vi "test_TCP_TCP Get Error Node.vi"(8 "error in (no error)":errorcluster, 11 "TestCase in":refnum<class "Ethernet Protocol Tests.lvclass">) -> (0 "error out":errorcluster, 3 "TestCase out":refnum<class "Ethernet Protocol Tests.lvclass">)   [LabVIEW 2019, in "Ethernet Protocol Tests.lvclass"]
uses:
  Ethernet Protocol Tests.lvclass
  TCP/TCP.lvclass
  <vilib>/addons/_JKI Toolkits/VI Tester/TestCase.llb/TestCase.lvclass
  C:/Program Files (x86)/National Instruments/LabVIEW 2019/vi.lib/addons/_JKI Toolkits/VI Tester/TestCase.llb/TestCase.lvclass
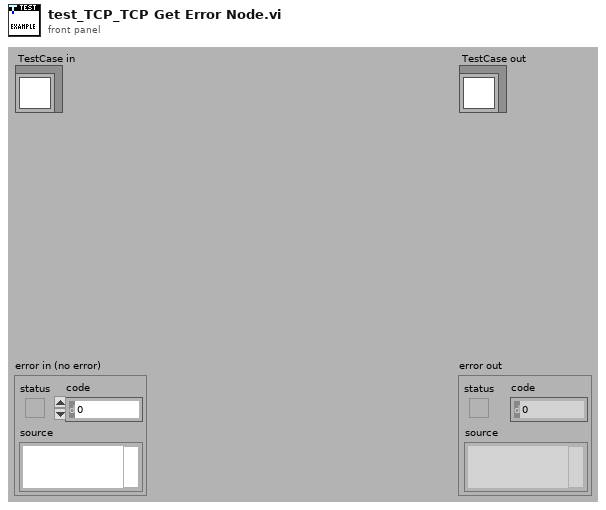
[diagram p1: front panel]
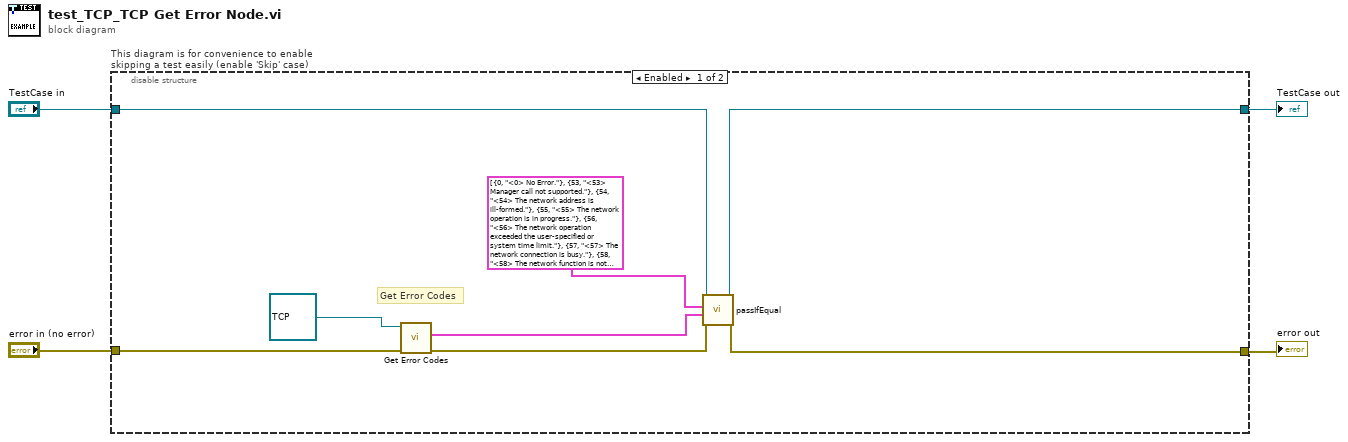
[diagram p0: block diagram]
diagram:
  n1 = disable-structure "This diagram is for convenience to enable skipping a test easily (enable 'Skip' case)" shown="Enabled" {
    disable-tunnel: "TestCase in" -> [w12 w16]
    disable-tunnel: [w11 w14] -> w1
    disable-tunnel: [w10 w15] -> w3
    disable-tunnel: "error in (no error)" -> [w8 w13]
    frame Enabled {
      # "Get Error Codes"
      n2 = call-dynamic "Get Error Codes.vi"("error in (no error)"=w8, "TCP in"=refnum<class "TCP.lvclass"> refnum ("Protocols.lvlib:TCP.lvclass")) -> ("error out"=w9:errorcluster, "Error Codes"=w5:cluster{"Code":i32, "String":string}[])  [unwired: 7 in, 1 out]
      n3 = call-dynamic "passIfEqual.vi"("error in (no error)"=w9, "y"=w5, "x"=cluster{"Code":i32, "String":string}[] [{"Code"=0, "String"="<0> No Error."}, {"Code"=53, "String"="<53> Manager call not supported."}, {"Code"=54, "String"="<54> The network address is ill-formed."}, {"Code"=55, "String"="<55> The network operation is in progress."}, {"Code"=56, "String"="<56> The network operation exceeded the user-specified or system time limit."}, {"Code"=57, "String"="<57> The network connection is busy."}, {"Code"=58, "String"="<58> The network function is not supported by the system."}, {"Code"=59, "String"="<59> The network is down, unreachable, or has been reset."}, {"Code"=60, "String"="<60> The specified port or network address is currently in use."}, {"Code"=61, "String"="<61> The system could not allocate the necessary memory."}, {"Code"=62, "String"="<62> The system caused the network connection to be aborted."}, {"Code"=63, "String"="<63> The network connection was refused by the server."}, {"Code"=64, "String"="<64> The network connection is not yet established."}, {"Code"=65, "String"="<65> The network connection is already established."}, {"Code"=66, "String"="<66> The network connection was closed by the peer."}, {"Code"=114, "String"="<114> Could not create TCP listener port because the port, service name, or net address conflict with a TCP listener that already exists."}, {"Code"=127, "String"="<127> The specified socket is not an IPv4 socket."}] ("Error Codes"), "TestCase in"=w12) -> ("error out"=w10:errorcluster, "TestCase out"=w11:refnum<class "Ethernet Protocol Tests.lvclass">)  [unwired: 6 in]
    }
    frame Disabled {
      # "skip test result while test is under development"
      n4 = call <vilib>:"skip.vi"("error in (no error)"=w13, "TestCase in"=w16) -> ("error out"=w15:errorcluster, "TestCase out"=w14:refnum<class "Ethernet Protocol Tests.lvclass">)  [unwired: 8 in]
    }
  }
  "error out" <- w3
  "TestCase out" <- w1
